vi "UpdateRobotStatus.vi"(0 "Operation Interface in":refnum<class "Operation Interface.lvclass">, 1 "Robot Status":T1, 5 "error in (no error)":errorcluster) -> (14 "Operation Interface out":refnum<class "Operation Interface.lvclass">, 15 "Robot Status Out":T1, 19 "error out":errorcluster)   [LabVIEW 2016, in "Operation Interface.lvclass"]
uses:
  Operation Interface.lvclass
  Universal Robot/RobotStatus.ctl
  Universal Robot/RobotMode.ctl
  Universal Robot/OperationalMode.ctl
  Universal Robot/SafetyStatus.ctl
  Operation Interface.lvclass/Operation Interface.ctl
  Universal Robot/Universal Robot.lvclass
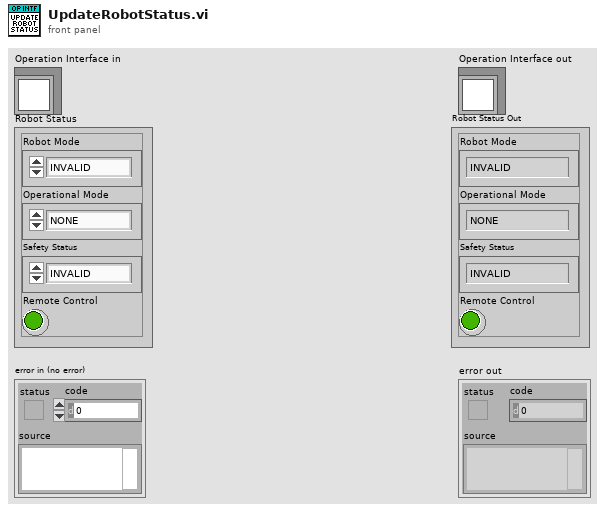
[diagram p1: front panel]
types:
  T1 = typedef "Universal Robot.lvclass/RobotStatus.ctl" = cluster{"Robot Mode":T2, "Operational Mode":T3, "Safety Status":T4, "Remote Control":bool}
  T2 = typedef "Universal Robot.lvclass/RobotMode.ctl" = enum16{"INVALID", "NO_CONTROLLER", "DISCONNECTED", "CONFIRM_SAFETY", "BOOTING", "POWER_OFF", "POWER_ON", "IDLE", "BACKDRIVE", "RUNNING"}
  T3 = typedef "Universal Robot.lvclass/OperationalMode.ctl" = enum16{"NONE", "MANUAL", "AUTOMATIC"}
  T4 = typedef "Universal Robot.lvclass/SafetyStatus.ctl" = enum16{"INVALID", "NORMAL", "REDUCED", "PROTECTIVE_STOP", "RECOVERY", "SAFEGAURD_STOP", "SYSTEM_EMERGENCY_STOP", "ROBOT_EMERGENCY_STOP", "VIOLATION", "FAULT", "AUTOMATIC_MODE_SAFEGAURD_STOP", "SYSTEM_THREE_POSITION_ENABLING_STOP"}
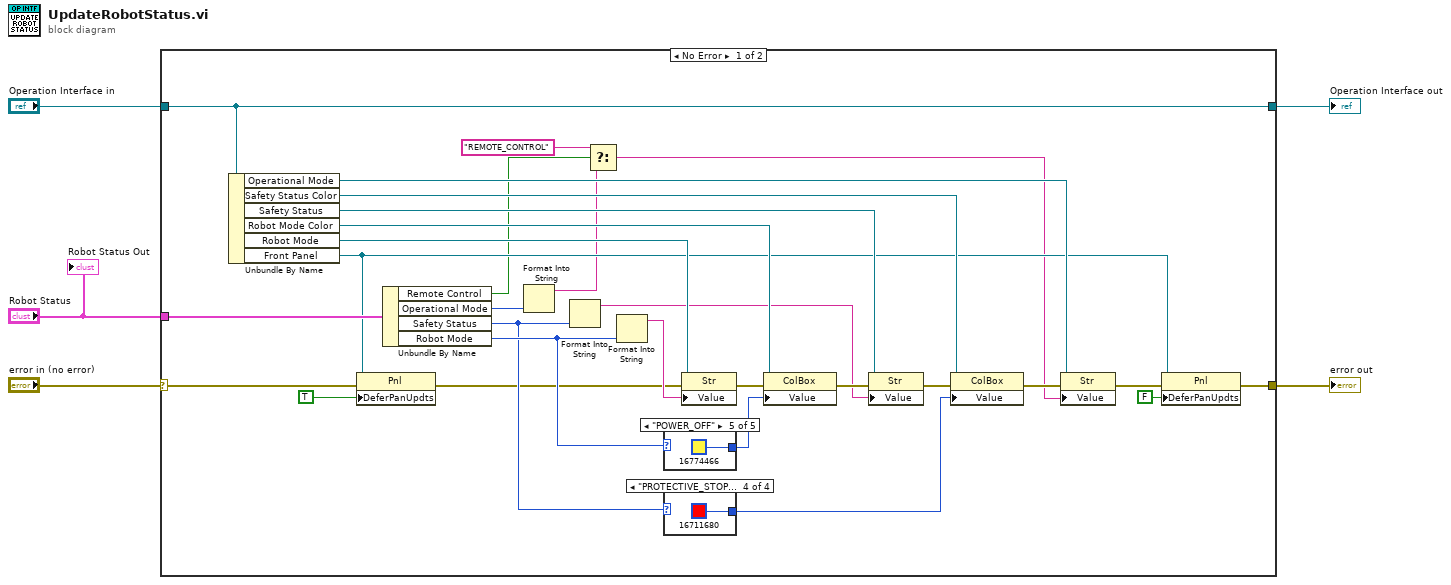
[diagram p0: block diagram]
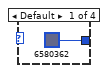
[diagram p2: hidden frame]
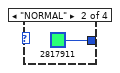
[diagram p3: hidden frame]
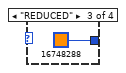
[diagram p4: hidden frame]
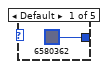
[diagram p5: hidden frame]
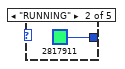
[diagram p6: hidden frame]
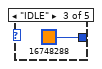
[diagram p7: hidden frame]
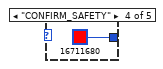
[diagram p8: hidden frame]
diagram:
  n1 = case shown="No Error" "error in (no error)" {
    selector: "error in (no error)" -> [w19 w45]
    tunnel: [w10 w45] -> w4
    tunnel: [w34 w44] -> w2
    tunnel: "Operation Interface in" -> [w34 w44]
    tunnel: "Robot Status" -> [w33 _]
    frame No Error {
      n2 = Unbundle By Name(w34) -> ("Operational Mode"=w14:refnum<vi>, "Safety Status Color"=w23:refnum<vi>, "Safety Status"=w25:refnum<vi>, "Robot Mode Color"=w28:refnum<vi>, "Robot Mode"=w32:refnum<vi>, "Front Panel"=w11:refnum<vi>)
      n3 = property class="Pnl"(reference=w11, error in=w19, "DeferPanUpdts"=TRUE ("Defer Panel Updates")) -> (error out=w18:errorcluster)  [unwired: 1 out]
      n4 = Unbundle By Name(w33) -> ("Remote Control"=w8:bool, "Operational Mode"=w16:T3, "Safety Status"=w22:T4, "Robot Mode"=w29:T2)
      n5 = Format Into String(w16) -> (resulting string=w9:string)  [unwired: 3 in, 1 out]
      n6 = Format Into String(w22) -> (resulting string=w20:string)  [unwired: 3 in, 1 out]
      n7 = Select(t="REMOTE_CONTROL", s=w8, f=w9) -> (s? t:f=w7:string)
      n8 = Format Into String(w29) -> (resulting string=w31:string)  [unwired: 3 in, 1 out]
      n9 = case shown="\"POWER_OFF\"" w29 {
        tunnel: [u32 6580362 u32 2817911 u32 16748288 u32 16711680 u32 16774466] -> w27
        frame Default {
        }
        frame "RUNNING" {
        }
        frame "IDLE" {
        }
        frame "CONFIRM_SAFETY" {
        }
        frame "POWER_OFF" {
        }
      }
      n10 = case shown="\"PROTECTIVE_STOP\", \"SAFEGAURD_STOP\"..\"FAULT\"" w22 {
        tunnel: [u32 6580362 u32 2817911 u32 16748288 u32 16711680] -> w21
        frame Default {
        }
        frame "NORMAL" {
        }
        frame "REDUCED" {
        }
        frame "PROTECTIVE_STOP", "SAFEGAURD_STOP".."FAULT" {
        }
      }
      n11 = property class="Str"(reference=w32, error in=w18, "Value"=w31) -> (error out=w30:errorcluster)  [unwired: 1 out]
      n12 = property class="ColBox"(reference=w28, error in=w30, "Value"=w27) -> (error out=w26:errorcluster)  [unwired: 1 out]
      n13 = property class="Str"(reference=w25, error in=w26, "Value"=w20) -> (error out=w24:errorcluster)  [unwired: 1 out]
      n14 = property class="ColBox"(reference=w23, error in=w24, "Value"=w21) -> (error out=w15:errorcluster)  [unwired: 1 out]
      n15 = property class="Str"(reference=w14, error in=w15, "Value"=w7) -> (error out=w12:errorcluster)  [unwired: 1 out]
      n16 = property class="Pnl"(reference=w11, error in=w12, "DeferPanUpdts"=FALSE ("Defer Panel Updates")) -> (error out=w10:errorcluster)  [unwired: 1 out]
    }
    frame Error {
    }
  }
  "error out" <- w4
  "Operation Interface out" <- w2
  "Robot Status Out" <- "Robot Status"
